vi "GUI_Bella_LaserTable_Frontend.vi"() -> ()   [LabVIEW 2020]
uses:
  Shared/GUI_Template/GUI_master/tcp_new_data_event.ctl
  Shared/GUI_Template/GUI_master/tcp new data cluster.ctl
  <vilib>/vision/Image Controls.llb/IMAQ Image.ctl
  <vilib>/ErrorRing/Error Ring.xnode
panel:
  in  "size1Y":dbl=20.0 caption="Size Y" min=0.0 max=0.0
  out "error out":errorcluster
  out "image::7":T1(plugin-control) caption="M1 Cam"
  out "image::8":T1(plugin-control) caption="M1 Cam"
  in  "image::6":T1(plugin-control) caption="M1 Cam"
  out "Display5":T1(plugin-control) caption="M1 Cam"
  in  "Target.X::5":dbl=0.001 caption="X" min=0.0 max=2000.0
  in  "Target.Y::5":dbl=0.001 caption="Y" min=0.0 max=2000.0
  in  "size5":dbl=20.0 caption="Size" min=0.0 max=0.0
  out "Display4":T1(plugin-control) caption="M1 Cam"
  in  "Target.X::4":dbl=0.001 caption="X" min=0.0 max=2000.0
  in  "Target.Y::4":dbl=0.001 caption="Y" min=0.0 max=2000.0
  in  "size4":dbl=20.0 caption="Size" min=0.0 max=0.0
  out "Display3":T1(plugin-control) caption="M1 Cam"
  in  "Target.X::3":dbl=0.001 caption="X" min=0.0 max=2000.0
  in  "Target.Y::3":dbl=0.001 caption="Y" min=0.0 max=2000.0
  in  "size3":dbl=20.0 caption="Size" min=0.0 max=0.0
  in  "Target.X::2":dbl=0.001 caption="X" min=0.0 max=2000.0
  in  "Target.Y::2":dbl=0.001 caption="Y" min=0.0 max=2000.0
  in  "size2":dbl=20.0 caption="Size" min=0.0 max=0.0
  out "Display2":T1(plugin-control) caption="M1 Cam"
  in  "roi::5":bool caption="Blank Button"
  in  "centroidx::5":dbl=0.001 caption="X" min=0.0 max=0.0
  in  "centroidy::5":dbl=0.001 caption="Y" min=0.0 max=0.0
  in  "trigger::5":bool caption="Blank Button"
  in  "exposure::5":dbl=0.001 caption="Exposure" min=3.8e-05 max=1.0 format="%_4p"
  in  "GUIdevice 5":string="CAM-LT-Tel3L1" caption="CAMERA 5"
  in  "roi::4":bool caption="Blank Button"
  in  "centroidx::4":dbl=0.001 caption="X" min=0.0 max=0.0
  in  "centroidy::4":dbl=0.001 caption="Y" min=0.0 max=0.0
  in  "trigger::4":bool caption="Blank Button"
  in  "exposure::4":dbl=0.001 caption="Exposure" min=3.8e-05 max=1.0 format="%_4p"
  in  "GUIdevice 4":string="CAM-LT-AMP2mode" caption="CAMERA 4"
  in  "roi::3":bool caption="Blank Button"
  in  "centroidx::3":dbl=0.001 caption="X" min=0.0 max=0.0
  in  "centroidy::3":dbl=0.001 caption="Y" min=0.0 max=0.0
  in  "trigger::3":bool caption="Blank Button"
  in  "exposure::3":dbl=0.001 caption="Exposure" min=3.8e-05 max=1.0 format="%_4p"
  in  "GUIdevice 3":string="CAM-LT-Clunker" caption="CAMERA 3"
  in  "roi::1":bool caption="Blank Button"
  in  "size1X":dbl=20.0 caption="Size X" min=0.0 max=0.0
  in  "Target.X::1":dbl=0.001 caption="X" min=0.0 max=2000.0
  in  "Target.Y::1":dbl=0.001 caption="Y" min=0.0 max=2000.0
  in  "centroidx::1":dbl=0.001 caption="X" min=0.0 max=0.0
  in  "centroidy::1":dbl=0.001 caption="Y" min=0.0 max=0.0
  in  "trigger::1":bool caption="Blank Button"
  in  "exposure::1":dbl=0.001 caption="Exposure" min=3.8e-05 max=1.0 format="%_4p"
  in  "GUIdevice 1":string="CAM-LT-DogLegMirror" caption="CAMERA 1"
  out "Display1":T1(plugin-control) caption="M1 Cam"
  in  "roi::2":bool caption="Blank Button"
  in  "centroidx::2":dbl=0.001 caption="X" min=0.0 max=0.0
  in  "centroidy::2":dbl=0.001 caption="Y" min=0.0 max=0.0
  in  "trigger::2":bool caption="Blank Button"
  in  "exposure::2":dbl=0.001 caption="Exposure" min=3.8e-05 max=1.0 format="%_4p"
  in  "GUIdevice 2":string="CAM-LT-Tel2" caption="CAMERA 2"
  out "image::5":T1(plugin-control) caption="M1 Cam"
  out "image::4":T1(plugin-control) caption="M1 Cam"
  in  "image::3":T1(plugin-control) caption="M1 Cam"
  out "image::2":T1(plugin-control) caption="M1 Cam"
  out "image::1":T1(plugin-control) caption="M1 Cam"
  out "tcp data event":T2
  in  "stop":bool
  out "error IO 2":errorcluster
  # "LASER TABLE GUI - 1"
  # "Target"
  # "Centroid"
  # "Centroid"
  # "Target"
  # "Target"
  # "Centroid"
  # "Centroid"
  # "Target"
  # "Centroid"
  # "Target"
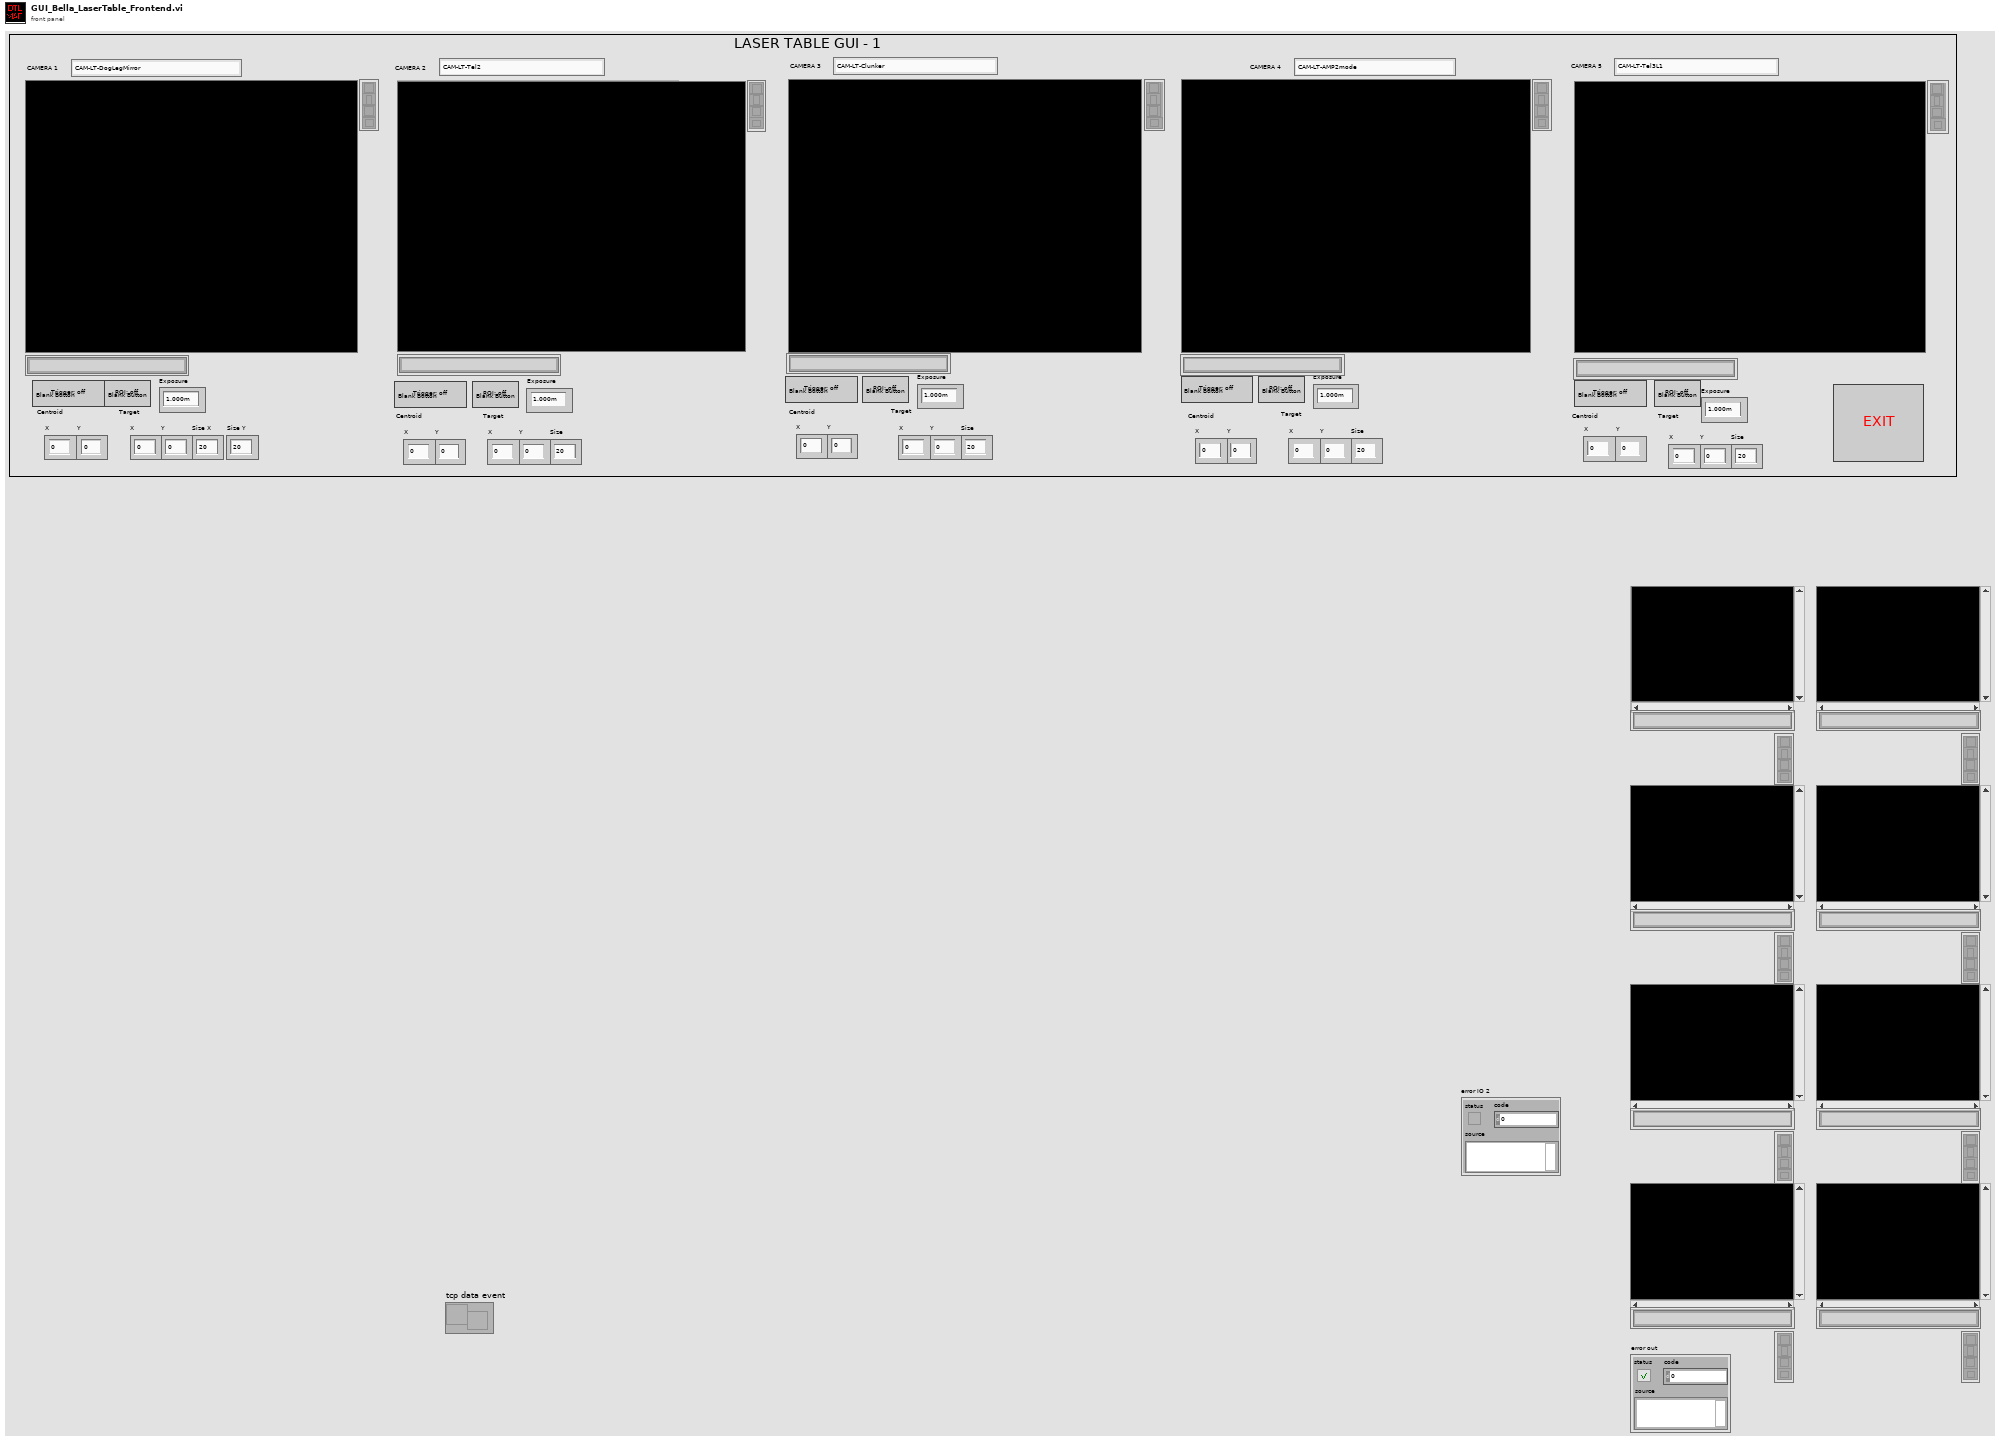
[diagram p1: front panel]
types:
  T1 = typedef "IMAQ Image.ctl" = refnum<image>
  T2 = typedef "tcp_new_data_event.ctl" = refnum<user-event>
  T3 = cluster{"Image1":T1, "Image2":T1, "Image3":T1, "Image4":T1, "Image5":T1, "Image6":T1, "Image7":T1, "Image8":T1}
  T4 = cluster{"Last update Cam1":u32, "Last update Cam2":u32, "Last update Cam3":u32, "Last update Cam4":u32, "Last update Cam5":u32, "Last update Cam6":u32, "Last update Cam7":u32, "Last update Cam8":u32}
  T5 = typedef "Image Type" = u32
  T6 = typedef "tcp new data cluster.ctl" = cluster{"EventEnum":enum16{"new data", "connection status update"}, "Device name":string}
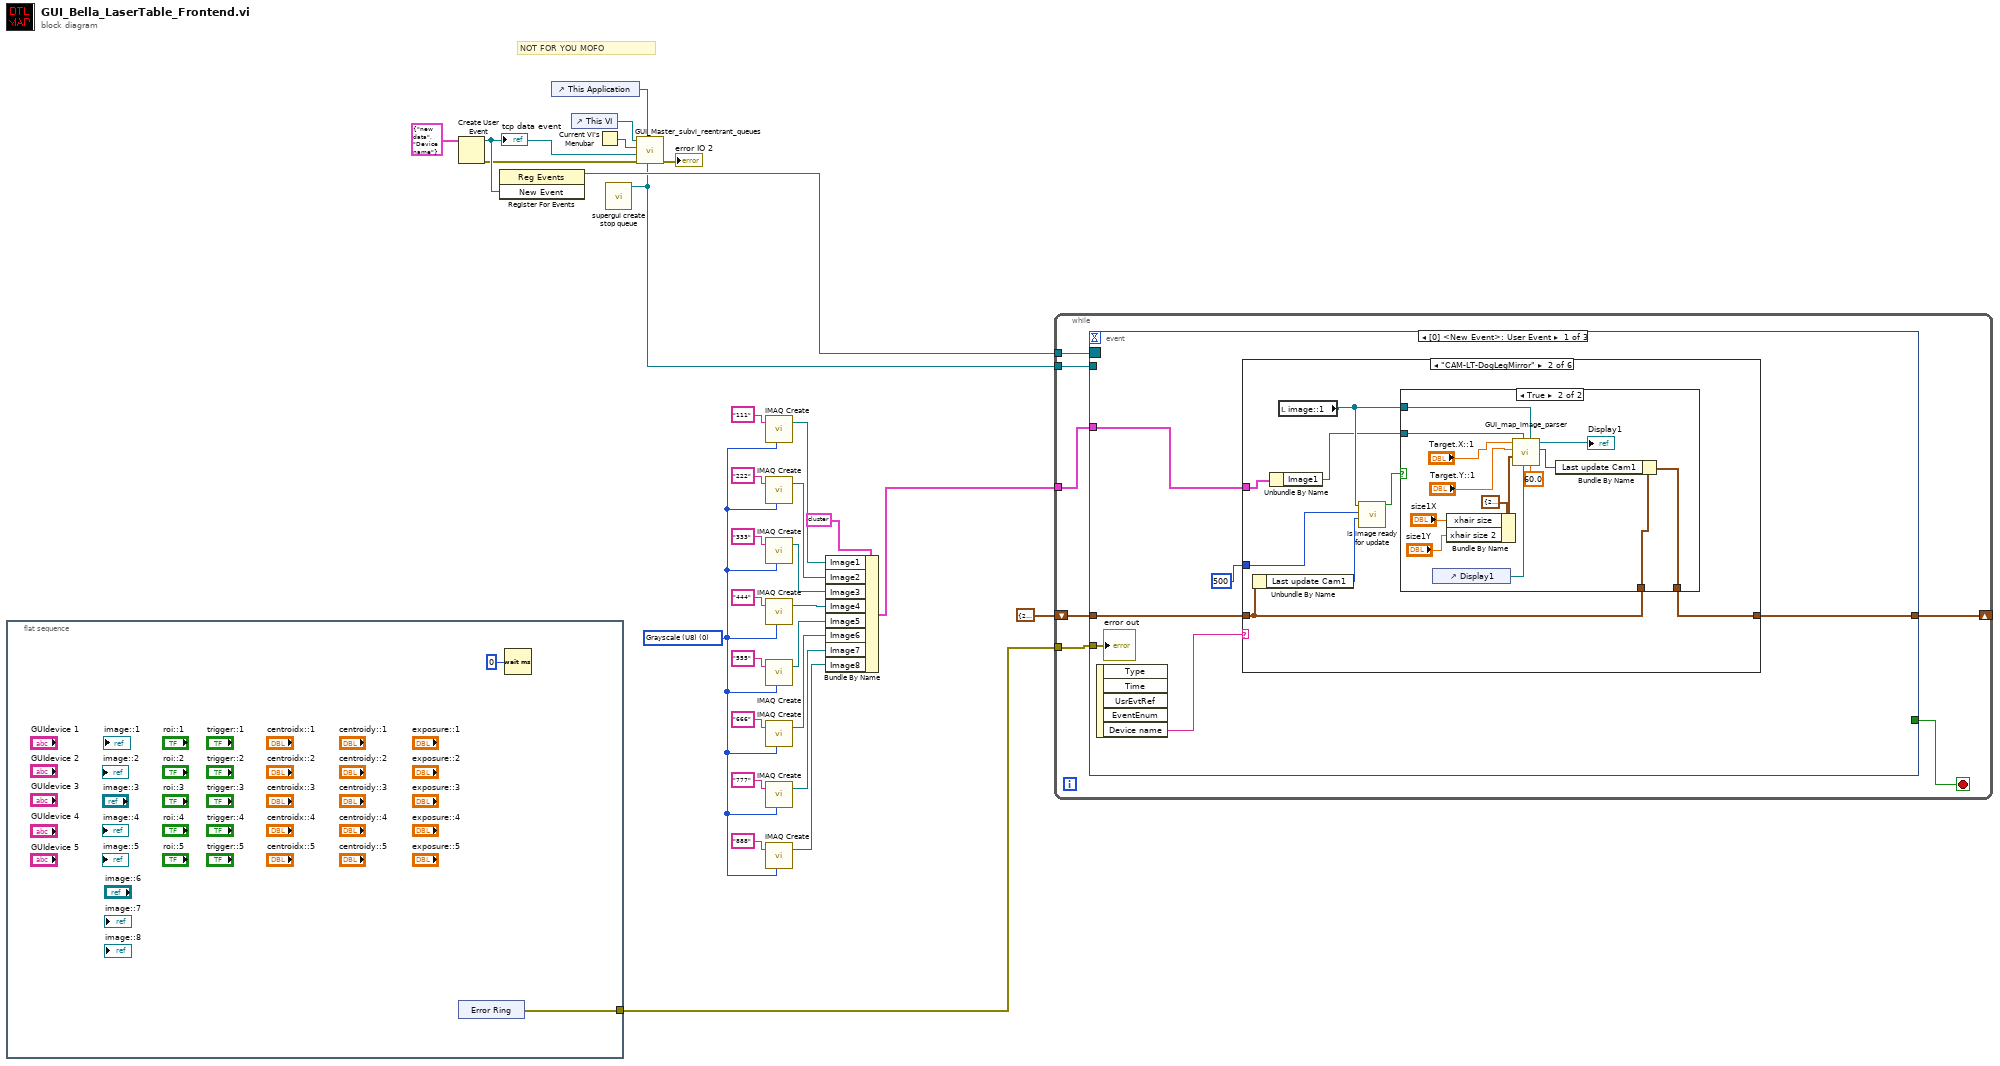
[diagram p0: block diagram]
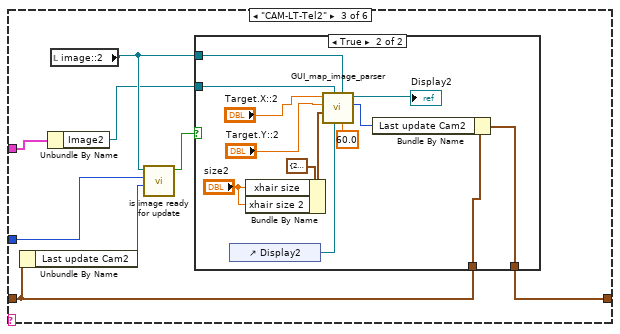
[diagram p4: hidden frame]
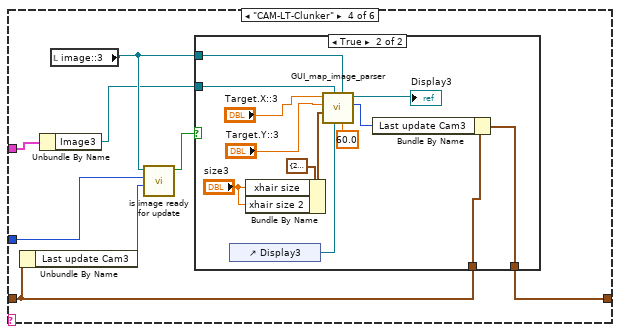
[diagram p6: hidden frame]
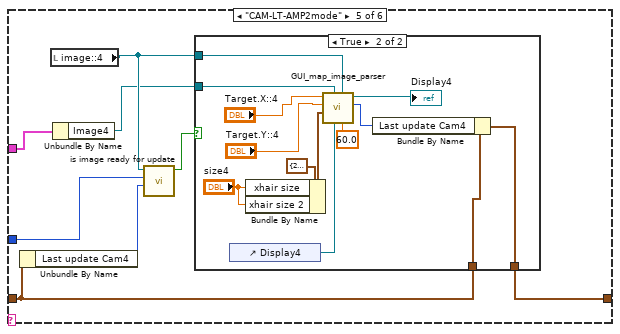
[diagram p8: hidden frame]
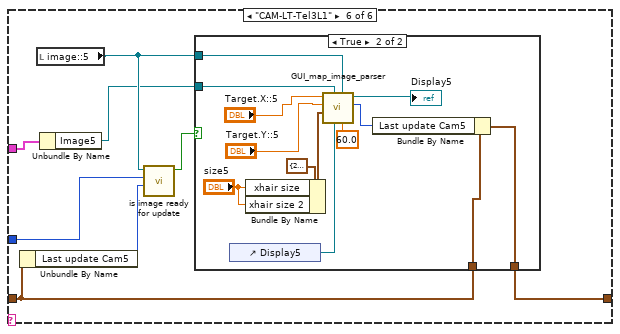
[diagram p10: hidden frame]
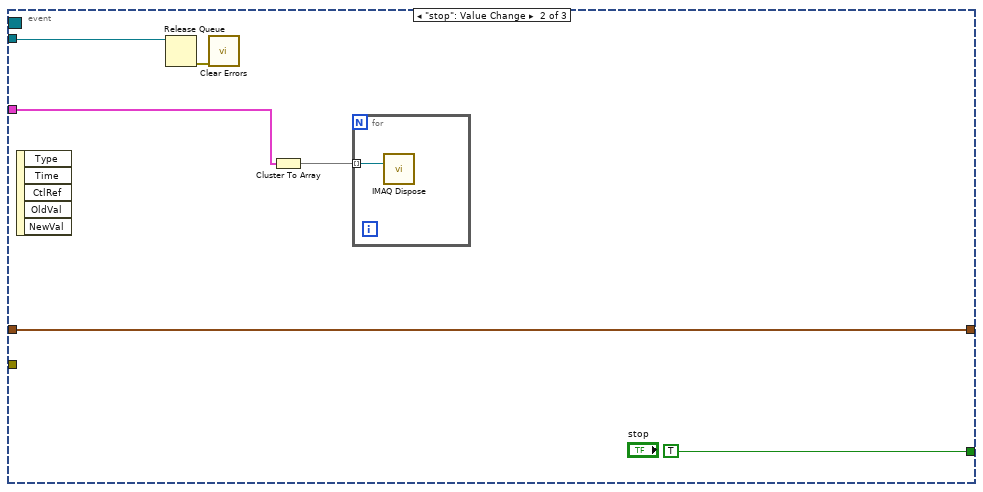
[diagram p12: hidden frame]
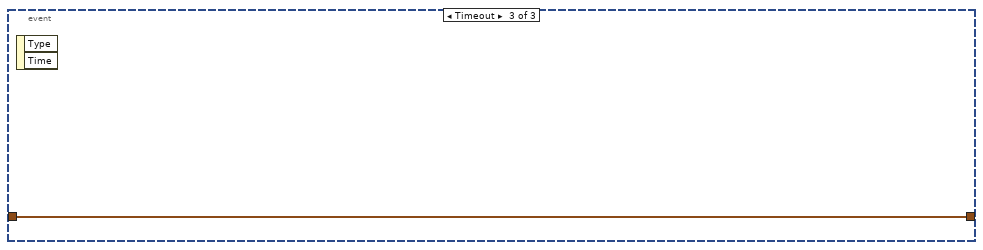
[diagram p13: hidden frame]
diagram:
  w12 = T5 0 items=["Grayscale (U8)", "Grayscale (I16)", "Grayscale (SGL)", "Complex (CSG)", "RGB (U32)", "HSL (U32)", "RGB (U64)", "Grayscale (U16)"] ("Image Type")
  # "NOT FOR YOU MOFO"
  n1 = flat-sequence {
    tunnel: [w32] -> w1
    frame #0 {
      n2 = xnode "Error Ring"() -> ("error out"=w32:errorcluster)
      n3 = Wait (ms)(milliseconds to wait=u32 0) -> ()  [unwired: 1 out]
    }
  }
  n4 = Create User Event(user event datatype=T6 {"EventEnum"=enum."new data", "Device name"="Device name"} ("New Event")) -> (user event=w29:refnum<user-event>, error out=w28:errorcluster)  [unwired: 1 in]
  "tcp data event" <- w29
  n5 = register-events(w29) -> (reference out=w24:refnum<event-registration>)  [unwired: 2 in, 1 out]
  n6 = control-ref of="This Application"() -> (w30:refnum<vi>)
  n7 = control-ref of="This VI"() -> (w25:refnum<vi>)
  n8 = Current VI's Menubar() -> (w26:refnum<k9>)
  n9 = call "supergui create stop queue.vi"() -> ("STOP Queue out"=w16:refnum<queue>)  [unwired: 11 in]
  n10 = call "GUI_Master_subvi_reentrant_queues.vi"("STOP Queue in"=w16, "This Application"=w30, "error in (no error)"=w28, "tcp data event"=w29, "Caller menu reference"=w26, "Caller VI ref"=w25) -> ("error out"=→"error IO 2":errorcluster)  [unwired: 5 in]
  n11 = call "IMAQ Create"("Image Name"="111", "Image Type"=w12) -> ("New Image"=w11:T1)  [unwired: 3 in, 1 out]
  n12 = call "IMAQ Create"("Image Name"="222", "Image Type"=w12) -> ("New Image"=w10:T1)  [unwired: 3 in, 1 out]
  n13 = call "IMAQ Create"("Image Name"="333", "Image Type"=w12) -> ("New Image"=w9:T1)  [unwired: 3 in, 1 out]
  n14 = call "IMAQ Create"("Image Name"="444", "Image Type"=w12) -> ("New Image"=w8:T1)  [unwired: 3 in, 1 out]
  n15 = call "IMAQ Create"("Image Name"="555", "Image Type"=w12) -> ("New Image"=w7:T1)  [unwired: 3 in, 1 out]
  n16 = call "IMAQ Create"("Image Name"="666", "Image Type"=w12) -> ("New Image"=w6:T1)  [unwired: 3 in, 1 out]
  n17 = call "IMAQ Create"("Image Name"="777", "Image Type"=w12) -> ("New Image"=w5:T1)  [unwired: 3 in, 1 out]
  n18 = call "IMAQ Create"("Image Name"="888", "Image Type"=w12) -> ("New Image"=w4:T1)  [unwired: 3 in, 1 out]
  n19 = Bundle By Name(cluster=T3 {"Image1"=refnum, "Image2"=refnum, "Image3"=refnum, "Image4"=refnum, "Image5"=refnum, "Image6"=refnum, "Image7"=refnum, "Image8"=refnum}, "Image1"=w11, "Image2"=w10, "Image3"=w9, "Image4"=w8, "Image5"=w7, "Image6"=w6, "Image7"=w5, "Image8"=w4) -> (w2:T3)
  n20 = while {
    tunnel: w24 -> [w39]
    shift-right: [w37] -> _
    shift-left: T4 {"Last update Cam1"=200, "Last update Cam2"=200, "Last update Cam3"=200, "Last update Cam4"=200, "Last update Cam5"=200, "Last update Cam6"=200, "Last update Cam7"=200, "Last update Cam8"=200} -> [w38]
    tunnel: w16 -> [w36]
    tunnel: w2 -> [w35]
    tunnel: w1 -> [w34]
    stop <- w40 stop-if-true
    n21 = event shown="[0] <New Event>: User Event" {
      selector: w39 -> [_ _ _]
      dyn-events: _ -> [_ _ _]
      timeout: _ -> [_ _ _]
      tunnel: [_ TRUE ("stop") _] -> w40
      tunnel: w38 -> [w45 w163 w166]
      tunnel: [w43 w163 w166] -> w37
      tunnel: w36 -> [_ w162 _]
      tunnel: w35 -> [w42 w160 _]
      tunnel: w34 -> [w41 _ _]
      event User Event {
        n22 = event-data() -> ("Device name"=w46:string)  [unwired: 1 in, 4 out]
        n23 = case shown="\"CAM-LT-DogLegMirror\"" w46 {
          tunnel: w45 -> [w47 w55 w78 w100 w122 w144]
          tunnel: u32 500 ("x-y") -> [_ w53 w76 w98 w120 w142]
          tunnel: [w47 w54 w77 w99 w121 w143] -> w43
          tunnel: w42 -> [_ w49 w72 w94 w116 w138]
          frame Default {
          }
          frame "CAM-LT-DogLegMirror" {
            n24 = Unbundle By Name(w55) -> ("Last update Cam1"=w52:u32)
            n25 = Unbundle By Name(w49) -> ("Image1"=w48:T1)
            n26 = local read "image::1"() -> (w50:T1)
            n27 = call "is image ready for update.vi"("Last update"=w52, "min time between updates"=w53, "image ref in"=w50) -> ("update image"=w51:bool)  [unwired: 8 in]
            n28 = case shown="True" w51 {
              tunnel: w55 -> [w56 w70]
              tunnel: [w56 w69] -> w54
              tunnel: w50 -> [_ w68]
              tunnel: w48 -> [_ w58]
              frame False {
              }
              frame True {
                n29 = control-ref of="Display1"() -> (w64:refnum<vi>)
                n30 = Bundle By Name(cluster=cluster{"xhair size":dbl, "xhair size 2":dbl} {"xhair size"=20.0, "xhair size 2"=20.0} ("size"), "xhair size"="size1X", "xhair size 2"="size1Y") -> (w59:cluster{"xhair size":dbl, "xhair size 2":dbl})
                n31 = call "GUI_map_image_parser.vi"("zoom#"=60.0, "Image Src"=w68, "Ctl Refnum"=w64, "Image Dst"=w58, "size"=w59, "target y"="Target.Y::1", "target x"="Target.X::1") -> ("ms timer out"=w63:u32, "Img out"=→"Display1":T1)  [unwired: 3 in]
                n32 = Bundle By Name(cluster=w70, "Last update Cam1"=w63) -> (w69:T4)
              }
            }
          }
          frame "CAM-LT-Tel2" {
            n33 = Unbundle By Name(w78) -> ("Last update Cam2"=w75:u32)
            n34 = Unbundle By Name(w72) -> ("Image2"=w71:T1)
            n35 = local read "image::2"() -> (w73:T1)
            n36 = call "is image ready for update.vi"("Last update"=w75, "min time between updates"=w76, "image ref in"=w73) -> ("update image"=w74:bool)  [unwired: 8 in]
            n37 = case shown="True" w74 {
              tunnel: w78 -> [w79 w92]
              tunnel: [w79 w91] -> w77
              tunnel: w73 -> [_ w90]
              tunnel: w71 -> [_ w80]
              frame False {
              }
              frame True {
                n38 = control-ref of="Display2"() -> (w86:refnum<vi>)
                n39 = Bundle By Name(cluster=cluster{"xhair size":dbl, "xhair size 2":dbl} {"xhair size"=20.0, "xhair size 2"=20.0} ("size"), "xhair size"="size2", "xhair size 2"="size2") -> (w81:cluster{"xhair size":dbl, "xhair size 2":dbl})
                n40 = call "GUI_map_image_parser.vi"("zoom#"=60.0, "Image Src"=w90, "Ctl Refnum"=w86, "Image Dst"=w80, "size"=w81, "target y"="Target.Y::2", "target x"="Target.X::2") -> ("ms timer out"=w85:u32, "Img out"=→"Display2":T1)  [unwired: 3 in]
                n41 = Bundle By Name(cluster=w92, "Last update Cam2"=w85) -> (w91:T4)
              }
            }
          }
          frame "CAM-LT-Clunker" {
            n42 = Unbundle By Name(w100) -> ("Last update Cam3"=w97:u32)
            n43 = Unbundle By Name(w94) -> ("Image3"=w93:T1)
            n44 = local read "image::3"() -> (w95:T1)
            n45 = call "is image ready for update.vi"("Last update"=w97, "min time between updates"=w98, "image ref in"=w95) -> ("update image"=w96:bool)  [unwired: 8 in]
            n46 = case shown="True" w96 {
              tunnel: w100 -> [w101 w114]
              tunnel: [w101 w113] -> w99
              tunnel: w95 -> [_ w112]
              tunnel: w93 -> [_ w102]
              frame False {
              }
              frame True {
                n47 = control-ref of="Display3"() -> (w108:refnum<vi>)
                n48 = Bundle By Name(cluster=cluster{"xhair size":dbl, "xhair size 2":dbl} {"xhair size"=20.0, "xhair size 2"=20.0} ("size"), "xhair size"="size3", "xhair size 2"="size3") -> (w103:cluster{"xhair size":dbl, "xhair size 2":dbl})
                n49 = call "GUI_map_image_parser.vi"("zoom#"=60.0, "Image Src"=w112, "Ctl Refnum"=w108, "Image Dst"=w102, "size"=w103, "target y"="Target.Y::3", "target x"="Target.X::3") -> ("ms timer out"=w107:u32, "Img out"=→"Display3":T1)  [unwired: 3 in]
                n50 = Bundle By Name(cluster=w114, "Last update Cam3"=w107) -> (w113:T4)
              }
            }
          }
          frame "CAM-LT-AMP2mode" {
            n51 = Unbundle By Name(w122) -> ("Last update Cam4"=w119:u32)
            n52 = local read "image::4"() -> (w117:T1)
            n53 = Unbundle By Name(w116) -> ("Image4"=w115:T1)
            n54 = call "is image ready for update.vi"("Last update"=w119, "min time between updates"=w120, "image ref in"=w117) -> ("update image"=w118:bool)  [unwired: 8 in]
            n55 = case shown="True" w118 {
              tunnel: w122 -> [w123 w136]
              tunnel: [w123 w135] -> w121
              tunnel: w117 -> [_ w134]
              tunnel: w115 -> [_ w124]
              frame False {
              }
              frame True {
                n56 = control-ref of="Display4"() -> (w130:refnum<vi>)
                n57 = Bundle By Name(cluster=cluster{"xhair size":dbl, "xhair size 2":dbl} {"xhair size"=20.0, "xhair size 2"=20.0} ("size"), "xhair size"="size4", "xhair size 2"="size4") -> (w125:cluster{"xhair size":dbl, "xhair size 2":dbl})
                n58 = call "GUI_map_image_parser.vi"("zoom#"=60.0, "Image Src"=w134, "Ctl Refnum"=w130, "Image Dst"=w124, "size"=w125, "target y"="Target.Y::4", "target x"="Target.X::4") -> ("ms timer out"=w129:u32, "Img out"=→"Display4":T1)  [unwired: 3 in]
                n59 = Bundle By Name(cluster=w136, "Last update Cam4"=w129) -> (w135:T4)
              }
            }
          }
          frame "CAM-LT-Tel3L1" {
            n60 = Unbundle By Name(w144) -> ("Last update Cam5"=w141:u32)
            n61 = local read "image::5"() -> (w139:T1)
            n62 = Unbundle By Name(w138) -> ("Image5"=w137:T1)
            n63 = call "is image ready for update.vi"("Last update"=w141, "min time between updates"=w142, "image ref in"=w139) -> ("update image"=w140:bool)  [unwired: 8 in]
            n64 = case shown="True" w140 {
              tunnel: w144 -> [w145 w158]
              tunnel: [w145 w157] -> w143
              tunnel: w139 -> [_ w156]
              tunnel: w137 -> [_ w146]
              frame False {
              }
              frame True {
                n65 = control-ref of="Display5"() -> (w152:refnum<vi>)
                n66 = Bundle By Name(cluster=cluster{"xhair size":dbl, "xhair size 2":dbl} {"xhair size"=20.0, "xhair size 2"=20.0} ("size"), "xhair size"="size5", "xhair size 2"="size5") -> (w147:cluster{"xhair size":dbl, "xhair size 2":dbl})
                n67 = call "GUI_map_image_parser.vi"("zoom#"=60.0, "Image Src"=w156, "Ctl Refnum"=w152, "Image Dst"=w146, "size"=w147, "target y"="Target.Y::5", "target x"="Target.X::5") -> ("ms timer out"=w151:u32, "Img out"=→"Display5":T1)  [unwired: 3 in]
                n68 = Bundle By Name(cluster=w158, "Last update Cam5"=w151) -> (w157:T4)
              }
            }
          }
        }
        "error out" <- w41
      }
      event "stop": Value Change {
        n69 = event-data() -> ()  [unwired: 1 in, 5 out]
        n70 = Release Queue(queue=w162) -> (error out=w161:errorcluster)  [unwired: 2 in, 2 out]
        n71 = call <vilib>:"Clear Errors.vi"("error in (no error)"=w161) -> ()  [unwired: 5 in, 2 out]
        n72 = Cluster To Array(cluster=w160) -> (array=w159:T1[])
        n73 = for {
          tunnel: w159 -> [w165] mode=indexing
          n74 = call "IMAQ Dispose"("Image"=w165) -> ()  [unwired: 5 in, 1 out]
        }
      }
      event Timeout {
        n75 = event-data() -> ()  [unwired: 1 in, 2 out]
      }
    }
  }
